vi "SelfTest-FlattenPackets.vi"() -> ()   [LabVIEW 2013, in "MQTT Server.lvlib" / "PacketCollection.lvclass"]
uses:
  PacketCollection.lvclass
  <vilib>/LabVIEW Open Source Project/MQTT Control Packets/Control Packets/ControlPacket/Control Packet Type -- enum.ctl
  <vilib>/LabVIEW Open Source Project/MQTT Control Packets/Control Packets/ControlPacket/QualityOfService -- enum.ctl
  <vilib>/LabVIEW Open Source Project/MQTT Control Packets/Control Packets/ControlPacket/ControlPacket.lvclass
  <vilib>/LabVIEW Open Source Project/MQTT Control Packets/Control Packets/PUBLISH/PUBLISH.lvclass
  PacketCollection.lvclass/PacketCollection.ctl
panel:
  out "Array":T1[](array[typedef])
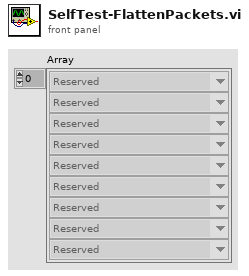
[diagram p1: front panel]
types:
  T1 = typedef "MQTT_Control_Packets.lvlib/ControlPacket.lvclass/Control Packet Type -- enum.ctl" = enum16{"Reserved", "CONNECT", "CONNACK", "PUBLISH", "PUBACK", "PUBREC", "PUBREL", "PUBCOMP", "SUBSCRIBE", "SUBACK", "UNSUBSCRIBE", "UNSUBACK", "PINGREQ", "PINGRESP", "DISCONNECT", "AUTH"}
  T2 = typedef "MQTT_Control_Packets.lvlib/ControlPacket.lvclass/QualityOfService -- enum.ctl" = enum16{"0 (At Most Once)", "1 (At Least Once)", "2 (Exactly Once)"}
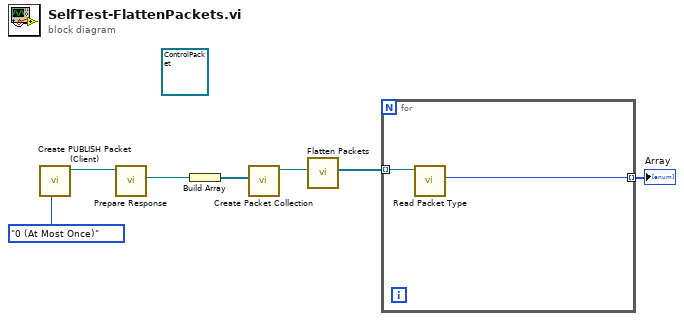
[diagram p0: block diagram]
diagram:
  (unwired) refnum<class "ControlPacket.lvclass"> refnum ("Incoming Packet")
  n1 = call <vilib>:"Create PUBLISH Packet (Client).vi"("QoS"=QualityOfService_--_enum."0 (At Most Once)") -> ("PUBLISH"=w3:refnum<class "PUBLISH.lvclass">)  [unwired: 7 in, 3 out]
  n2 = call-dynamic "Prepare Response.vi"("PUBLISH in"=w3) -> ("ControlPacket response"=w1:refnum<class "ControlPacket.lvclass">)  [unwired: 7 in, 3 out]
  n3 = Build Array(w1) -> (w5:refnum<class "ControlPacket.lvclass">[])
  n4 = call "Create Packet Collection.vi"("Packets"=w5) -> ("PacketCollection"=w4:refnum<class "PacketCollection.lvclass">)  [unwired: 10 in]
  n5 = call "Flatten Packets.vi"("Incoming Packet"=w4) -> ("Packets"=w7:refnum<class "ControlPacket.lvclass">[])  [unwired: 10 in]
  n6 = for {
    tunnel: w7 -> [w9] mode=indexing
    tunnel: [w8] -> w6 mode=indexing
    n7 = call <vilib>:"Read Packet Type.vi"("ControlPacket in"=w9) -> ("Control Packet Type"=w8:T1)  [unwired: 9 in, 1 out]
  }
  "Array" <- w6
